vi "Teleop.vi"(10 "Match Info":T4={"Autonomous Elapsed Seconds"=0.0, "TeleOp Elapsed Seconds"=0.0, "Disabled Elapsed Seconds"=0.0, "Visited Autonomous"=FALSE, "Visited TeleOp"=FALSE, "Visited Disabled"=FALSE, "Autonomous Settings"={"Autonomous Style"=enum."Independent", "VI Refnum"=refnum}}, 11 "Call Context":T5) -> ()   [LabVIEW 2020]
doc: "This VI is called for each TeleOp packet received from the DS where the robot is not disabled. It is often used to read from the joysticks and update I/O or to update setpoints for timed control loops. It should complete and return within 20 milliseconds or it may miss DS packets."
uses:
  <vilib>/Rock Robotics/WPI/DriverStation/WPI_DriverStationDerivedRobotMode.ctl
  <vilib>/Rock Robotics/WPI/DriverStation/WPI_DriverStationMatch Info.ctl
  <vilib>/Rock Robotics/WPI/ThirdParty/Phoenix-LabVIEW/Motor Controller/Controls/CTRE_Phoenix_MotorControl_ControlMode.ctl
  <vilib>/Rock Robotics/WPI/Utilities/WPI_GetSetVariantRefNum.vi
  TitanLib/Lib/Piston Toggle.vi
  <vilib>/Rock Robotics/Network Tables/NT Write Boolean Array.vi
  <vilib>/Rock Robotics/Network Tables/NT Write Numeric Array.vi
  <vilib>/Rock Robotics/WPI/Solenoid/WPI_SolenoidSetEnum.vi
  globals.vi
  <vilib>/Rock Robotics/WPI/ThirdParty/Phoenix-LabVIEW/Motor Controller/Get/CTRE_Phoenix_MotorController_GetSelectedSensorData.vi
  <vilib>/addons/control/pid/pid.llb/PID (DBL).vi
  <vilib>/addons/control/pid/NI_PID_pid.lvlib
  TitanLib/Lib/TitanLib.lvlib
  <vilib>/Rock Robotics/WPI/ThirdParty/Phoenix-LabVIEW/Motor Controller/Get/CTRE_Phoenix_MotorController_GetSupplyAndStatorCurrent_Enhanced.vi
  TitanLib/Lib/RPMToRawUnits-2048-CPR.vi
  TitanLib/Lib/RawUnitsToRPM-2048-CPR.vi
panel:
  in  "magazine power":dbl=1.0
  in  "kicker power":dbl=-1.0
  in  "intake power":dbl=1.0
  out "UpperSensor":bool
  out "LowerSensor":bool
  in  "Flywheel PIDF Constants":T1={"Set Constants"=FALSE, "P"=0.1, "I"=0.001, "D"=0.0, "F"=0.0461, "I Zone"=1000.0, "Cruise Velocity"=0, "Acceleration"=0, "Percent Deadband"=0.0}
  out "Raw Units":i32
  in  "Setpoint RPM":dbl=7000.0
  out "Shooter Motor Current":T2(graph)
  out "Rpm":cluster{"RPM":dbl, "Setpoint RPM":dbl}(graph)
  out "Waveform Chart":cluster{dbl, dbl}(graph)
  in  "Zero Encoders":bool
  in  "Climber PIDF":T1={"Set Constants"=FALSE, "P"=0.45, "I"=0.0, "D"=0.0, "F"=0.0, "I Zone"=0.0, "Cruise Velocity"=20000, "Acceleration"=20000, "Percent Deadband"=0.7}
  in  "Climber Manual Power":dbl
  in  "Climber Manual Override?":bool=TRUE
  in  "Climber Up Pos":dbl=-9.82
  in  "Climber Down Pos":dbl=-0.5
  out "Loop Time (ms)":u32(graph)
  in  "POV Power":dbl
  in  "Turn Speed":dbl=0.7
  out "Gyro PID Out":dbl
  in  "Gyro PID Deadband":dbl=0.2
  in  "Gyro PID Constants":T3={"proportional gain (Kc)"=0.035, "integral time (Ti, min)"=0.0, "derivative time (Td, min)"=0.0} {"derivative time (Td, min)" format="%.3f"; "integral time (Ti, min)" format="%.3f"; "proportional gain (Kc)" format="%.3f"}
  in  "Field Oriented Rotation? (Theta)":bool
  in  "Field Oriented Translation? (x/y)":bool=TRUE
  in  "Joystick Deadband":dbl=0.07
  # "Other"
  # "Misc."
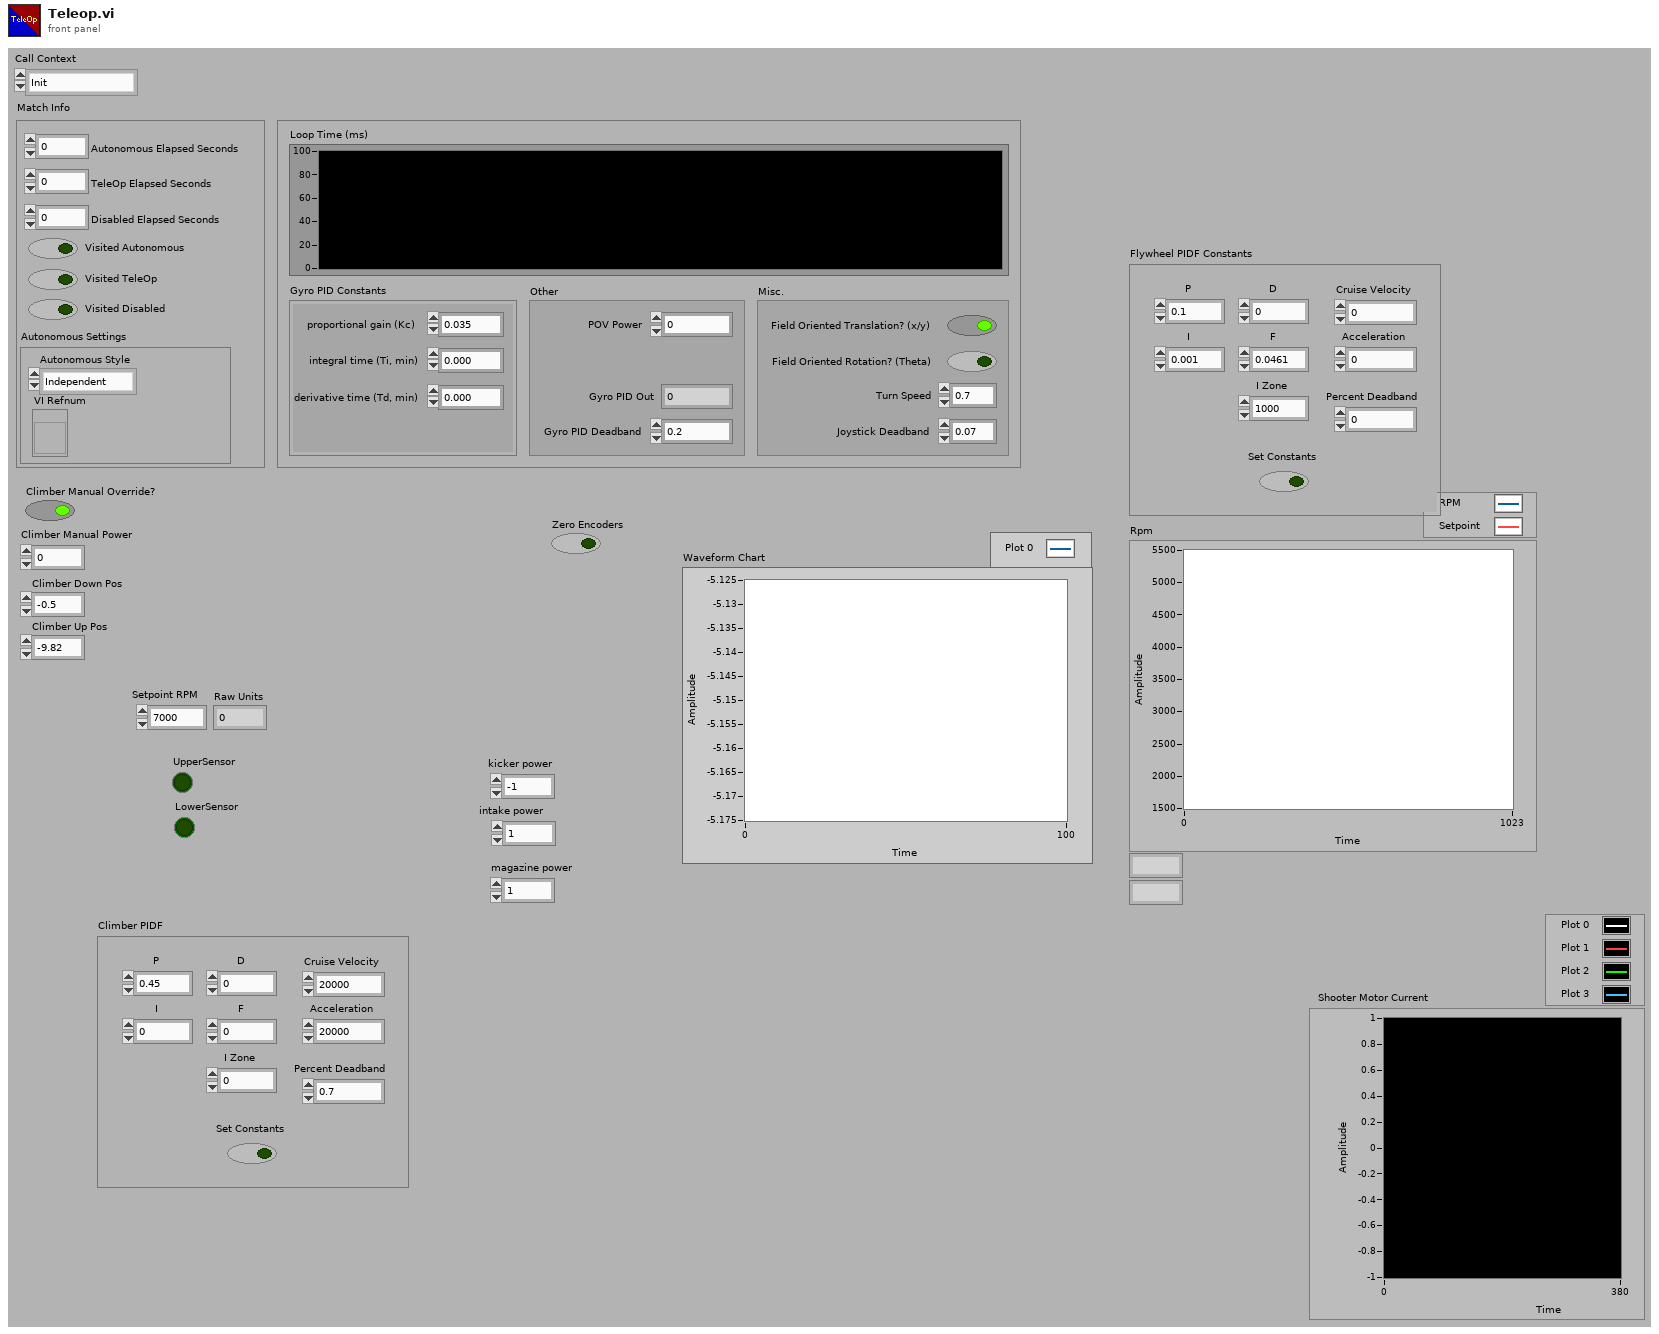
[diagram p1: front panel]
types:
  T1 = cluster{"Set Constants":bool, "P":dbl, "I":dbl, "D":dbl, "F":dbl, "I Zone":dbl, "Cruise Velocity":i32, "Acceleration":i32, "Percent Deadband":dbl}
  T2 = cluster{"Supply Current":dbl, "Stator Current":dbl, "Supply Current":dbl, "Stator Current":dbl}
  T3 = cluster{"proportional gain (Kc)":dbl, "integral time (Ti, min)":dbl, "derivative time (Td, min)":dbl}
  T4 = typedef "WPI_DriverStationMatch Info.ctl" = cluster{"Autonomous Elapsed Seconds":dbl, "TeleOp Elapsed Seconds":dbl, "Disabled Elapsed Seconds":dbl, "Visited Autonomous":bool, "Visited TeleOp":bool, "Visited Disabled":bool, "Autonomous Settings":cluster{"Autonomous Style":enum16{"Iterative", "Independent"}, "VI Refnum":refnum<vi>}}
  T5 = typedef "WPI_DriverStationDerivedRobotMode.ctl" = enum16{"Init", "Execute", "Stop"}
  T6 = typedef "CTRE_Phoenix_MotorControl_ControlMode.ctl" = u16
  T7 = typedef "WPI_JoystickDevRef.ctl" = cluster{"Device":T8}
  T8 = typedef "WPI_JoystickDeviceEnum.ctl" = enum16{"USB 0", "USB 1", "USB 2", "USB 3", "USB 4", "USB 5"}
  T9 = typedef "WPI_SolenoidValue.ctl" = enum16{"Off", "On", "Forward", "Reverse"}
  T10 = typedef "WPI_SolenoidDevRef.ctl" = cluster{"DevStatus":errorcluster, "Pneumatics Control Module":u8, "Forward Solenoid Channel":T11, "Reverse Solenoid Channel":T11}
  T11 = typedef "WPI_SolenoidChannel.ctl" = enum8{"Solenoid 0", "Solenoid 1", "Solenoid 2", "Solenoid 3", "Solenoid 4", "Solenoid 5", "Solenoid 6", "Solenoid 7", "Solenoid 8", "Solenoid 9", "Solenoid 10", "Solenoid 11", "Solenoid 12", "Solenoid 13", "Solenoid 14", "Solenoid 15", "Invalid"}
  T12 = typedef "WPI_MotorControlDeviceRef.ctl" = cluster{"DeviceStatus":errorcluster, "Type":T13, "PWM":cluster{"PWM Channel":T14, "DeadBand":T15}, "CAN":cluster{"Device Number":u8, "SetOutput VI Ref":variant, "GetOutput VI Ref":variant, "Enable VI Ref":variant, "Disable VI Ref":variant, "Data":variant}, "Invert":bool, "DIO PWM":cluster{"PWM \"Enable\" Channel":T14, "DIOChannel":T16, "PWM Rate":dbl}}
  T13 = typedef "WPI_MotorControlType.ctl" = enum16{"PWM", "CAN", "DIO PWM"}
  T14 = typedef "FPGA_DIOPWMChannel.ctl" = enum8{"PWM 0", "PWM 1", "PWM 2", "PWM 3", "PWM 4", "PWM 5", "PWM 6", "PWM 7", "PWM 8", "PWM 9", "PWM MXP 0", "PWM MXP 1", "PWM MXP 2", "PWM MXP 3", "PWM MXP 4", "PWM MXP 5", "PWM MXP 6", "PWM MXP 7", "PWM MXP 8", "PWM MXP 9", "Invalid"}
  T15 = typedef "WPI_PWMDeadband.ctl" = cluster{"Name":string, "maxPositivePwm":i32, "minPositivePwm":i32, "centerPwm":i32, "maxNegativePwm":i32, "minNegativePwm":i32, "angularRange":u16}
  T16 = typedef "FPGA_DIOChannel.ctl" = enum8{"DIO 0", "DIO 1", "DIO 2", "DIO 3", "DIO 4", "DIO 5", "DIO 6", "DIO 7", "DIO 8", "DIO 9", "DIO MXP 0", "DIO MXP 1", "DIO MXP 2", "DIO MXP 3", "DIO MXP 4", "DIO MXP 5", "DIO MXP 6", "DIO MXP 7", "DIO MXP 8", "DIO MXP 9", "DIO MXP 10", "DIO MXP 11", "DIO MXP 12", "DIO MXP 13", "DIO MXP 14", "DIO MXP 15", "SPI Port CS1", "SPI Port CS2", "SPI Port CS3", "SPI Port MISO", "SPI Port MOSI", "Invalid"}
  T17 = typedef "WPI_DigitalInputDevRef.ctl" = cluster{"DevStatus":errorcluster, "DIO Channel":T16}
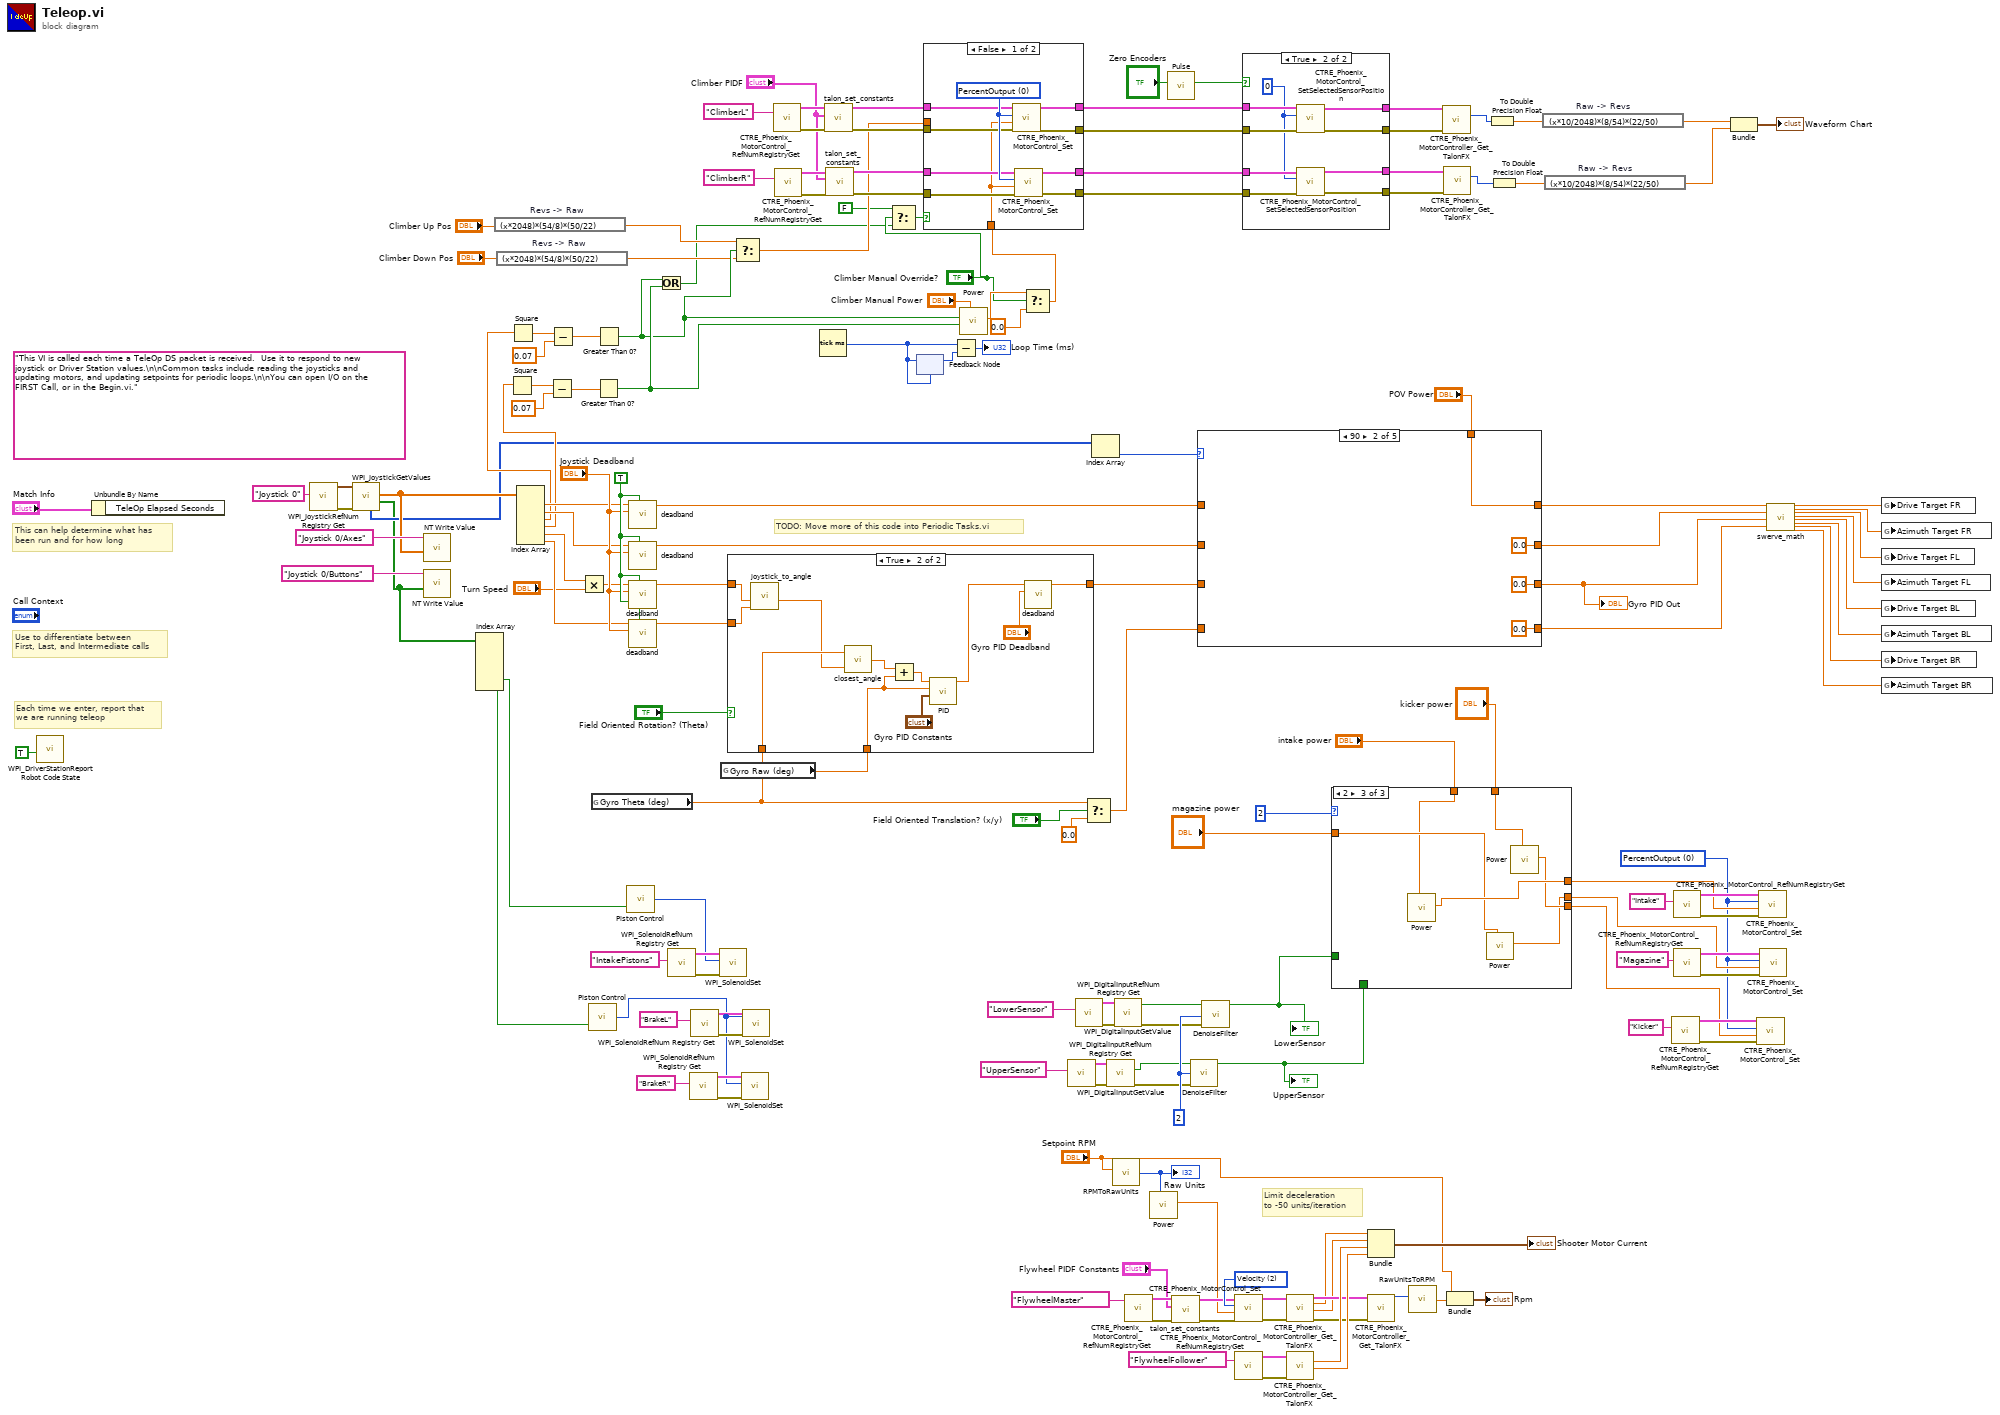
[diagram p0: block diagram]
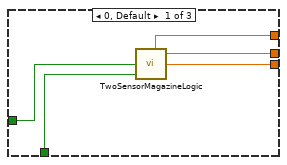
[diagram p2: hidden frame]
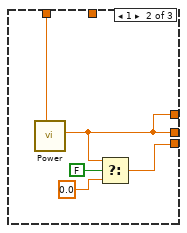
[diagram p3: hidden frame]
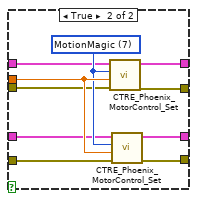
[diagram p5: hidden frame]
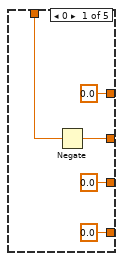
[diagram p6: hidden frame]
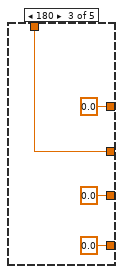
[diagram p7: hidden frame]
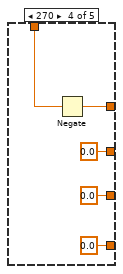
[diagram p8: hidden frame]
diagram:
  w7 = T6 0 items=["PercentOutput"=0, "Position"=1, "Velocity"=2, "Current"=3, "Follower"=5, "MotionProfile"=6, "MotionMagic"=7, "MotionProfileArc"=10, "Disabled"=15] ("Control Mode")
  w29 = T6 2 items=["PercentOutput"=0, "Position"=1, "Velocity"=2, "Current"=3, "Follower"=5, "MotionProfile"=6, "MotionMagic"=7, "MotionProfileArc"=10, "Disabled"=15] ("Control Mode")
  w48 = 2 ("Filter Level")
  w155 = TRUE ("Square Input?")
  (unwired) "This VI is called each time a TeleOp DS packet is received.  Use it to respond to new joystick or Driver Station values.\n\nCommon tasks include reading the joysticks and updating motors, and updating setpoints for periodic loops.\n\nYou can open I/O on the FIRST Call, or in the Begin.vi."
  # "Limit deceleration\nto -50 units/iteration"
  # "TODO: Move more of this code into Periodic Tasks.vi"
  # "Each time we enter, report that\nwe are running teleop"
  # "Use to differentiate between\nFirst, Last, and Intermediate calls"
  # "This can help determine what has\nbeen run and for how long"
  n1 = call <vilib>:"WPI_DriverStationReport Robot Code State.vi"("TeleOp"=TRUE ("Autonomous")) -> ()  [unwired: 10 in, 1 out]
  n2 = Unbundle By Name("Match Info") -> ()  [unwired: 1 out]
  n3 = call <vilib>:"WPI_JoystickRefNum Registry Get.vi"("refnum name"="Joystick 0") -> ("error out"=w158:errorcluster, "JoystickDevRef"=w163:T7)  [unwired: 1 in, 8 out]
  n4 = call <vilib>:"WPI_JoystickGetValues.vi"("error in (no error)"=w158, "JoystickDevRef"=w163) -> ("Buttons"=w107:bool[], "Axes"=w159:dbl[], "POVs"=w108:i16[])  [unwired: 5 in, 2 out]
  n5 = call-poly <vilib>:"NT Write Value.vi"("Numeric Array"=w159, "Name"="Joystick 0/Axes") -> ()  [unwired: 9 in, 1 out]
  n6 = call-poly <vilib>:"NT Write Value.vi"("Boolean Array"=w107, "Name"="Joystick 0/Buttons") -> ()  [unwired: 9 in, 1 out]
  n7 = Index Array(array=w107) -> (element #5=w106:bool, element #6=w101:bool)  [unwired: 6 in, 4 out]
  n8 = expression code="(x*2048)*(54/8)*(50/22)" "Revs -> Raw"("Climber Up Pos") -> (w64:dbl)
  n9 = expression code="(x*2048)*(54/8)*(50/22)" "Revs -> Raw"("Climber Down Pos") -> (w65:dbl)
  n10 = Index Array(array=w159) -> (element #1=w151:dbl, element #2=w150:dbl, element #3=w111:dbl, element #4=w110:dbl, element #5=w124:dbl, element #6=w149:dbl)  [unwired: 6 in]
  n11 = Square(x=w110) -> (x^2=w112:dbl)
  n12 = Square(x=w111) -> (x^2=w117:dbl)
  n13 = Subtract(x=w112, y=0.07 ("x")) -> (x-y=w114:dbl)
  n14 = Subtract(x=w117, y=0.07 ("x")) -> (x-y=w115:dbl)
  n15 = Multiply(x=w124, y="Turn Speed") -> (x*y=w139:dbl)
  n16 = call-poly "Piston Control.vi"("Input"=w101) -> ("Output"=w94:T9)  [unwired: 1 in]
  n17 = global read "globals.vi" "Gyro Theta (deg)"() -> (w128:dbl)
  n18 = Greater Than 0?(x=w114) -> (x > 0?=w67:bool)
  n19 = Greater Than 0?(x=w115) -> (x > 0?=w66:bool)
  n20 = call-poly "Piston Control.vi"("Input"=w106) -> ("Output"=w102:T9)  [unwired: 1 in]
  n21 = call "deadband.vi"("Square Input?"=w155, "Deadband"="Joystick Deadband", "In"=w151) -> ("Out"=w134:dbl)  [unwired: 8 in]
  n22 = call "deadband.vi"("Square Input?"=w155, "Deadband"="Joystick Deadband", "In"=w150) -> ("Out"=w136:dbl)  [unwired: 8 in]
  n23 = call "deadband.vi"("Square Input?"=w155, "Deadband"="Joystick Deadband", "In"=w139) -> ("Out"=w148:dbl)  [unwired: 8 in]
  n24 = call "deadband.vi"("Square Input?"=w155, "Deadband"="Joystick Deadband", "In"=w149) -> ("Out"=w154:dbl)  [unwired: 8 in]
  n25 = Or(x=w66, y=w67) -> (x .or. y?=w57:bool)
  n26 = call <vilib>:"WPI_SolenoidRefNum Registry Get.vi"("refnum name"="IntakePistons") -> ("error out"=w105:errorcluster, "SolenoidDevRef"=w104:T10)  [unwired: 9 in]
  n27 = call <vilib>:"WPI_SolenoidRefNum Registry Get.vi"("refnum name"="BrakeR") -> ("error out"=w98:errorcluster, "SolenoidDevRef"=w97:T10)  [unwired: 9 in]
  n28 = call <vilib>:"WPI_SolenoidRefNum Registry Get.vi"("refnum name"="BrakeL") -> ("error out"=w99:errorcluster, "SolenoidDevRef"=w100:T10)  [unwired: 9 in]
  n29 = call-poly <vilib>:"WPI_SolenoidSet.vi"("error in (no error)"=w105, "Value"=w102, "SolenoidDevRef"=w104) -> ()  [unwired: 7 in, 2 out]
  n30 = global read "globals.vi" "Gyro Raw (deg)"() -> (w129:dbl)
  n31 = case shown="True" "Field Oriented Rotation? (Theta)" {
    tunnel: w148 -> [w166 w171]
    tunnel: [w166 w173] -> w138
    tunnel: w154 -> [_ w170]
    tunnel: w128 -> [_ w176]
    tunnel: w129 -> [_ w168]
    frame False {
    }
    frame True {
      n32 = call "joystick_to_angle.vi"("y"=w170, "x"=w171) -> ("Theta"=w169:dbl)  [unwired: 9 in]
      n33 = call "closest_angle.vi"("b"=w169, "a"=w176) -> ("dir"=w175:dbl)
      n34 = Add(x=w175, y=w168) -> (x+y=w172:dbl)
      n35 = call-poly <vilib>:"PID.vi"("PID gains"="Gyro PID Constants", "process variable"=w168, "setpoint"=w172) -> ("output"=w174:dbl)  [unwired: 7 in, 1 out]
      n36 = call "deadband.vi"("Deadband"="Gyro PID Deadband", "In"=w174) -> ("Out"=w173:dbl)  [unwired: 9 in]
    }
  }
  n37 = Select(t=w64, s=w66, f=w65) -> (s? t:f=w63:dbl)
  n38 = call-poly <vilib>:"WPI_SolenoidSet.vi"("error in (no error)"=w98, "Value"=w94, "SolenoidDevRef"=w97) -> ()  [unwired: 7 in, 2 out]
  n39 = call-poly <vilib>:"WPI_SolenoidSet.vi"("error in (no error)"=w99, "Value"=w94, "SolenoidDevRef"=w100) -> ()  [unwired: 7 in, 2 out]
  n40 = call <vilib>:"CTRE_Phoenix_MotorControl_RefNumRegistryGet.vi"("refnum name"="ClimberL") -> ("error out"=w92:errorcluster, "PhoenixMotorControlDevRef"=w93:T12)  [unwired: 9 in]
  n41 = call <vilib>:"CTRE_Phoenix_MotorControl_RefNumRegistryGet.vi"("refnum name"="ClimberR") -> ("error out"=w90:errorcluster, "PhoenixMotorControlDevRef"=w91:T12)  [unwired: 9 in]
  n42 = Tick Count (ms)() -> (millisecond timer value=w125:u32)
  n43 = call "talon_set_constants.vi"("error in"=w92, "Constants"="Climber PIDF", "PhoenixMotorControlDevRef"=w93) -> ("error out"=w87:errorcluster, "PhoenixMotorControlDevRef"=w86:T12)  [unwired: 7 in]
  n44 = call "talon_set_constants.vi"("error in"=w90, "Constants"="Climber PIDF", "PhoenixMotorControlDevRef"=w91) -> ("error out"=w89:errorcluster, "PhoenixMotorControlDevRef"=w88:T12)  [unwired: 7 in]
  n45 = Select(t=FALSE, s="Climber Manual Override?", f=w57) -> (s? t:f=w59:bool)
  n46 = feedback #1(w125) -> (w127:u32)
  n47 = feedback-in #1(w125) -> ()
  n48 = Subtract(x=w125, y=w127) -> (x-y=→"Loop Time (ms)":u32)
  n49 = call "Power.vi"("Positive Power"="Climber Manual Power", "Negative"=w67, "Positive"=w66) -> ("Output"=w62:dbl)  [unwired: 8 in]
  n50 = Select(t=w62, s="Climber Manual Override?", f=0.0 ("Output")) -> (s? t:f=w60:dbl)
  n51 = case shown="False" w59 {
    tunnel: w63 -> [_ w197]
    tunnel: w86 -> [w186 w195]
    tunnel: w88 -> [w184 w194]
    tunnel: w89 -> [w183 w193]
    tunnel: w87 -> [w185 w192]
    tunnel: w60 -> [w182 _]
    tunnel: [w181 w191] -> w84
    tunnel: [w180 w190] -> w83
    tunnel: [w179 w189] -> w82
    tunnel: [w178 w188] -> w81
    frame False {
      w187 = T6 0 items=["PercentOutput"=0, "Position"=1, "Velocity"=2, "Current"=3, "Follower"=5, "MotionProfile"=6, "MotionMagic"=7, "MotionProfileArc"=10, "Disabled"=15] ("Control Mode")
      n52 = call <vilib>:"CTRE_Phoenix_MotorControl_Set.vi"("error in (no error)"=w185, "Output"=w182, "Control Mode"=w187, "PhoenixMotorControlDevRef"=w186) -> ("error out"=w180:errorcluster, "PhoenixMotorControlDevRef"=w181:T12)  [unwired: 6 in]
      n53 = call <vilib>:"CTRE_Phoenix_MotorControl_Set.vi"("error in (no error)"=w183, "Output"=w182, "Control Mode"=w187, "PhoenixMotorControlDevRef"=w184) -> ("error out"=w178:errorcluster, "PhoenixMotorControlDevRef"=w179:T12)  [unwired: 6 in]
    }
    frame True {
      w196 = T6 7 items=["PercentOutput"=0, "Position"=1, "Velocity"=2, "Current"=3, "Follower"=5, "MotionProfile"=6, "MotionMagic"=7, "MotionProfileArc"=10, "Disabled"=15] ("Control Mode")
      n54 = call <vilib>:"CTRE_Phoenix_MotorControl_Set.vi"("error in (no error)"=w192, "Output"=w197, "Control Mode"=w196, "PhoenixMotorControlDevRef"=w195) -> ("error out"=w190:errorcluster, "PhoenixMotorControlDevRef"=w191:T12)  [unwired: 6 in]
      n55 = call <vilib>:"CTRE_Phoenix_MotorControl_Set.vi"("error in (no error)"=w193, "Output"=w197, "Control Mode"=w196, "PhoenixMotorControlDevRef"=w194) -> ("error out"=w188:errorcluster, "PhoenixMotorControlDevRef"=w189:T12)  [unwired: 6 in]
    }
  }
  n56 = call <vilib>:"WPI_DigitalInputRefNum Registry Get.vi"("refnum name"="UpperSensor") -> ("error out"=w54:errorcluster, "DigitalInputDevRef"=w55:T17)  [unwired: 9 in]
  n57 = call <vilib>:"WPI_DigitalInputRefNum Registry Get.vi"("refnum name"="LowerSensor") -> ("error out"=w51:errorcluster, "DigitalInputDevRef"=w50:T17)  [unwired: 9 in]
  n58 = Select(t=w128, s="Field Oriented Translation? (x/y)", f=0.0) -> (s? t:f=w131:dbl)
  n59 = Index Array(array=w108) -> (element=w133:i16)  [unwired: 1 in]
  n60 = call <vilib>:"WPI_DigitalInputGetValue.vi"("error in (no error)"=w54, "DigitalInputDevRef"=w55) -> ("error out"=w32:errorcluster, "Value"=w47:bool)  [unwired: 7 in, 1 out]
  n61 = call-poly "RPMToRawUnits.vi"("RPM"="Setpoint RPM") -> ("Raw Units"=w17:i32)  [unwired: 3 in]
  "Raw Units" <- w17
  n62 = call <vilib>:"WPI_DigitalInputGetValue.vi"("error in (no error)"=w51, "DigitalInputDevRef"=w50) -> ("error out"=w33:errorcluster, "Value"=w49:bool)  [unwired: 7 in, 1 out]
  n63 = call <vilib>:"CTRE_Phoenix_MotorControl_RefNumRegistryGet.vi"("refnum name"="FlywheelMaster") -> ("error out"=w11:errorcluster, "PhoenixMotorControlDevRef"=w12:T12)  [unwired: 9 in]
  n64 = call "Power.vi"("Positive Power"=w17) -> ("Output"=w2:dbl)  [unwired: 10 in]
  n65 = call "Pulse.vi"("Input"="Zero Encoders") -> ("Output"=w80:bool)  [unwired: 10 in]
  n66 = call "talon_set_constants.vi"("error in"=w11, "Constants"="Flywheel PIDF Constants", "PhoenixMotorControlDevRef"=w12) -> ("error out"=w9:errorcluster, "PhoenixMotorControlDevRef"=w10:T12)  [unwired: 7 in]
  n67 = call "DenoiseFIlter.vi"("error in (no error)"=w32, "Filter Level"=w48, "Signal Input"=w47) -> ("Signal Output"=w6:bool)  [unwired: 2 out]
  "UpperSensor" <- w6
  n68 = case shown="90" w133 {
    tunnel: [0.0 ("Out") 0.0 ("Out") 0.0 ("Out") 0.0 ("Out") w219] -> w122
    tunnel: w138 -> [_ _ _ _ w219]
    tunnel: [w200 0.0 ("Out") w209 0.0 ("Out") w218] -> w137
    tunnel: w136 -> [_ _ _ _ w218]
    tunnel: [0.0 ("Out") w206 0.0 ("Out") w211 w217] -> w135
    tunnel: w134 -> [_ _ _ _ w217]
    tunnel: "POV Power" -> [w201 w206 w209 w214 _]
    tunnel: [0.0 ("f") 0.0 ("f") 0.0 ("f") 0.0 ("f") w216] -> w130
    tunnel: w131 -> [_ _ _ _ w216]
    frame 0 {
      n69 = Negate(x=w201) -> (-x=w200:dbl)
    }
    frame 90 {
    }
    frame 180 {
    }
    frame 270 {
      n70 = Negate(x=w214) -> (-x=w211:dbl)
    }
    frame -1, Default {
    }
  }
  "Gyro PID Out" <- w122
  n71 = call "DenoiseFIlter.vi"("error in (no error)"=w33, "Filter Level"=w48, "Signal Input"=w49) -> ("Signal Output"=w46:bool)  [unwired: 2 out]
  "LowerSensor" <- w46
  n72 = call <vilib>:"CTRE_Phoenix_MotorControl_Set.vi"("error in (no error)"=w9, "Output"=w2, "Control Mode"=w29, "PhoenixMotorControlDevRef"=w10) -> ("error out"=w20:errorcluster, "PhoenixMotorControlDevRef"=w21:T12)  [unwired: 6 in]
  n73 = call <vilib>:"CTRE_Phoenix_MotorControl_RefNumRegistryGet.vi"("refnum name"="FlywheelFollower") -> ("error out"=w18:errorcluster, "PhoenixMotorControlDevRef"=w19:T12)  [unwired: 9 in]
  n74 = case shown="True" w80 {
    tunnel: w84 -> [w223 w232]
    tunnel: w83 -> [w222 w231]
    tunnel: w82 -> [w221 w230]
    tunnel: w81 -> [w220 w229]
    tunnel: [w223 w227] -> w78
    tunnel: [w222 w226] -> w77
    tunnel: [w221 w225] -> w76
    tunnel: [w220 w224] -> w75
    frame False {
    }
    frame True {
      w228 = 0 ("New Sensor Position")
      n75 = call <vilib>:"CTRE_Phoenix_MotorControl_SetSelectedSensorPosition.vi"("error in (no error)"=w231, "New Sensor Position"=w228, "PhoenixMotorControlDevRef"=w232) -> ("error out"=w226:errorcluster, "PhoenixMotorControlDevRef"=w227:T12)  [unwired: 7 in]
      n76 = call <vilib>:"CTRE_Phoenix_MotorControl_SetSelectedSensorPosition.vi"("error in (no error)"=w229, "New Sensor Position"=w228, "PhoenixMotorControlDevRef"=w230) -> ("error out"=w224:errorcluster, "PhoenixMotorControlDevRef"=w225:T12)  [unwired: 7 in]
    }
  }
  n77 = call-poly <vilib>:"CTRE_Phoenix_MotorController_Get_TalonFX.vi"("PhoenixMotorControlDevRef"=w21, "error in"=w20) -> ("PhoenixMotorControlDevRef"=w26:T12, "Supply Current"=w24:dbl, "Stator Current"=w23:dbl, "error out"=w25:errorcluster)  [unwired: 10 in]
  n78 = call-poly <vilib>:"CTRE_Phoenix_MotorController_Get_TalonFX.vi"("PhoenixMotorControlDevRef"=w19, "error in"=w18) -> ("Supply Current"=w28:dbl, "Stator Current"=w27:dbl)  [unwired: 10 in, 2 out]
  n79 = case shown="2" 2 {
    tunnel: w6 -> [w237 _ _]
    tunnel: w46 -> [w236 _ _]
    tunnel: [w235 w242 w248] -> w36
    tunnel: [w234 w242 w244] -> w35
    tunnel: [w233 w240 w246] -> w34
    tunnel: "intake power" -> [_ w239 w243]
    tunnel: "kicker power" -> [_ _ w247]
    tunnel: "magazine power" -> [_ _ w245]
    frame 0, Default {
      n80 = call "TwoSensorMagazineLogic.vi"("Intake Side Sensor"=w236, "Outtake Side Sensor"=w237) -> ("Intake Motors"=w235:dbl, "Magazine Motors"=w234:dbl, "Kicker Motors"=w233:dbl)  [unwired: 3 in, 2 out]
    }
    frame 1 {
      n81 = call "Power.vi"("Positive Power"=w239) -> ("Output"=w242:dbl)  [unwired: 10 in]
      n82 = Select(t=w242, s=FALSE, f=0.0) -> (s? t:f=w240:dbl)
    }
    frame 2 {
      n83 = call "Power.vi"("Positive Power"=w243) -> ("Output"=w248:dbl)  [unwired: 10 in]
      n84 = call "Power.vi"("Positive Power"=w245) -> ("Output"=w244:dbl)  [unwired: 10 in]
      n85 = call "Power.vi"("Positive Power"=w247) -> ("Output"=w246:dbl)  [unwired: 10 in]
    }
  }
  n86 = Bundle("Supply Current"=w24, "Stator Current"=w23, "Supply Current"=w28, "Stator Current"=w27) -> (→"Shooter Motor Current":T2)  [unwired: 1 in]
  n87 = call-poly <vilib>:"CTRE_Phoenix_MotorController_Get_TalonFX.vi"("PhoenixMotorControlDevRef"=w26, "error in"=w25) -> ("Velocity (Raw Sensor Units per 100 ms)"=w16:i32)  [unwired: 10 in, 3 out]
  n88 = call-poly "RawUnitsToRPM.vi"("Raw Units"=w16) -> ("RPM"=w15:dbl)  [unwired: 3 in]
  n89 = call-poly <vilib>:"CTRE_Phoenix_MotorController_Get_TalonFX.vi"("PhoenixMotorControlDevRef"=w78, "error in"=w77) -> ("Position (Raw Sensor Units)"=w70:i32)  [unwired: 10 in, 3 out]
  n90 = call-poly <vilib>:"CTRE_Phoenix_MotorController_Get_TalonFX.vi"("PhoenixMotorControlDevRef"=w76, "error in"=w75) -> ("Position (Raw Sensor Units)"=w69:i32)  [unwired: 10 in, 3 out]
  n91 = Bundle("RPM"=w15, "Setpoint RPM"="Setpoint RPM") -> (→"Rpm":cluster{"RPM":dbl, "Setpoint RPM":dbl})  [unwired: 1 in]
  n92 = To Double Precision Float(number=w70) -> (double precision float=w73:dbl)
  n93 = To Double Precision Float(number=w69) -> (double precision float=w74:dbl)
  n94 = expression code="(x*10/2048)*(8/54)*(22/50)" "Raw -> Revs"(w73) -> (w72:dbl)
  n95 = expression code="(x*10/2048)*(8/54)*(22/50)" "Raw -> Revs"(w74) -> (w71:dbl)
  n96 = call <vilib>:"CTRE_Phoenix_MotorControl_RefNumRegistryGet.vi"("refnum name"="Kicker") -> ("error out"=w43:errorcluster, "PhoenixMotorControlDevRef"=w42:T12)  [unwired: 9 in]
  n97 = call <vilib>:"CTRE_Phoenix_MotorControl_RefNumRegistryGet.vi"("refnum name"="Intake") -> ("error out"=w45:errorcluster, "PhoenixMotorControlDevRef"=w44:T12)  [unwired: 9 in]
  n98 = call <vilib>:"CTRE_Phoenix_MotorControl_RefNumRegistryGet.vi"("refnum name"="Magazine") -> ("error out"=w40:errorcluster, "PhoenixMotorControlDevRef"=w41:T12)  [unwired: 9 in]
  n99 = Bundle(w72, w71) -> (→"Waveform Chart":cluster{dbl, dbl})  [unwired: 1 in]
  n100 = call <vilib>:"CTRE_Phoenix_MotorControl_Set.vi"("error in (no error)"=w43, "Output"=w34, "Control Mode"=w7, "PhoenixMotorControlDevRef"=w42) -> ()  [unwired: 6 in, 2 out]
  n101 = call <vilib>:"CTRE_Phoenix_MotorControl_Set.vi"("error in (no error)"=w45, "Output"=w36, "Control Mode"=w7, "PhoenixMotorControlDevRef"=w44) -> ()  [unwired: 6 in, 2 out]
  n102 = call <vilib>:"CTRE_Phoenix_MotorControl_Set.vi"("error in (no error)"=w40, "Output"=w35, "Control Mode"=w7, "PhoenixMotorControlDevRef"=w41) -> ()  [unwired: 6 in, 2 out]
  n103 = call "swerve_math.vi"("Strafe"=w135, "Forwards"=w137, "Rotate"=w122, "Gyro"=w130) -> ("Drive FR"=w147:dbl, "Azimuth FR"=w146:dbl, "Drive FL"=w145:dbl, "Azimuth FL"=w144:dbl, "Drive BL"=w143:dbl, "Azimuth BL"=w142:dbl, "Drive BR"=w141:dbl, "Azimuth BR"=w140:dbl)  [unwired: 16 in]
  n104 = global write "globals.vi" "Drive Target FR"(w147) -> ()
  n105 = global write "globals.vi" "Azimuth Target FR"(w146) -> ()
  n106 = global write "globals.vi" "Drive Target FL"(w145) -> ()
  n107 = global write "globals.vi" "Azimuth Target FL"(w144) -> ()
  n108 = global write "globals.vi" "Drive Target BL"(w143) -> ()
  n109 = global write "globals.vi" "Azimuth Target BL"(w142) -> ()
  n110 = global write "globals.vi" "Drive Target BR"(w141) -> ()
  n111 = global write "globals.vi" "Azimuth Target BR"(w140) -> ()
